vi "Clear.vi"(8 "error in (no error)":errorcluster, 11 "Renderer":refnum<class "Renderer.lvclass">) -> (0 "error out":errorcluster)   [LabVIEW 2021, in "Renderer.lvclass"]
uses:
  Renderer.lvclass
  Renderer.lvclass/Renderer.ctl
  LabSDL2/Source/Libraries/LibSDL2 Wrapper/LibSDL2.lvlib
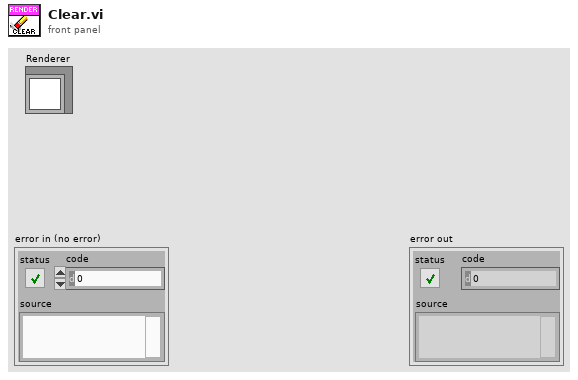
[diagram p1: front panel]
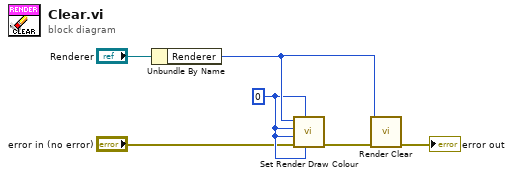
[diagram p0: block diagram]
diagram:
  w4 = u8 0 ("A")
  n1 = Unbundle By Name("Renderer") -> ("Renderer"=w6:u32)
  n2 = call "Set Render Draw Colour.vi"("B"=w4, "A"=w4, "error in (no error)"="error in (no error)", "G"=w4, "R"=w4, "Renderer Pointer"=w6) -> ("error out"=w5:errorcluster)  [unwired: 4 in, 1 out]
  n3 = call "Render Clear.vi"("error in"=w5, "Renderer Pointer"=w6) -> ("error out"=→"error out":errorcluster)  [unwired: 8 in, 1 out]
